vi "Initialize Instrument.vi"(8 "error in (no error)":errorcluster, 10 "Instr Resource Str":string, 11 "NI DMM.lvclass in":refnum<class "NI DMM.lvclass">) -> (0 "error out":errorcluster, 3 "NI DMM.lvclass out":refnum<class "NI DMM.lvclass">)   [LabVIEW 2011, in "NI DMM.lvclass"]
uses:
  NI DMM.lvclass
  NI DMM.lvclass/NI DMM.ctl
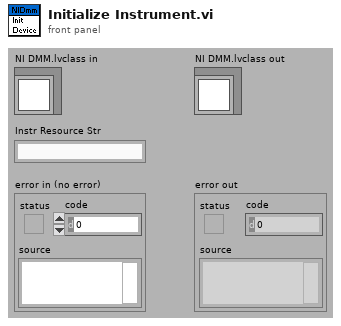
[diagram p1: front panel]
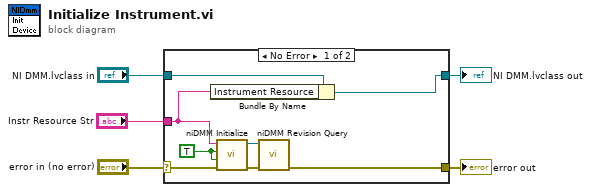
[diagram p0: block diagram]
diagram:
  n1 = case shown="No Error" "error in (no error)" {
    selector: "error in (no error)" -> [w9 w15]
    tunnel: [w11 w15] -> w5
    tunnel: "Instr Resource Str" -> [w6 _]
    tunnel: "NI DMM.lvclass in" -> [w8 w14]
    tunnel: [w7 w14] -> w4
    frame No Error {
      w13 = TRUE ("ID Query? (T: Yes)")
      n2 = Bundle By Name(cluster=w8, "Instrument Resource"=w6) -> (w7:refnum<class "NI DMM.lvclass">)
      n3 = call <instrlib>:"niDMM Initialize.vi"("error in (no error)"=w9, "Reset"=w13, "ID Query"=w13, "Instrument Descriptor"=w6) -> ("error out"=w12:errorcluster, "instrument handle out"=w10:refnum<k15>)  [unwired: 6 out]
      n4 = call <instrlib>:"niDMM Revision Query.vi"("error in (no error)"=w12, "instrument handle"=w10) -> ("error out"=w11:errorcluster)  [unwired: 9 out]
    }
    frame Error {
    }
  }
  "error out" <- w5
  "NI DMM.lvclass out" <- w4
